vi "Execute_Circle_v1.vi"(0 "Resolution":i32=20, 1 "Speed":i32, 2 "x-disp":sgl[](array[numeric]), 3 "y-disp":sgl[](array[numeric]), 4 "GPIB Address":u8=6 max=100) -> (5 "x-position":i32, 6 "y-position":i32, 7 "Status":bool)   [LabVIEW 2010]
uses:
  <vilib>/express/express arith-compare/Formula/XNode/ExpressFormulaBlockNode.xnode
panel:
  out "XY Graph":T1(graph)
  in  "y-disp read":i32[](array[numeric])
  in  "x-disp read":i32[](array[numeric])
  # "Inputs"
  # "Outputs"
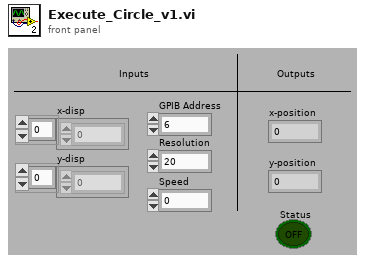
[diagram p1: front panel]
types:
  T1 = cluster{"x-disp read":i32[], "y-disp read":i32[]}
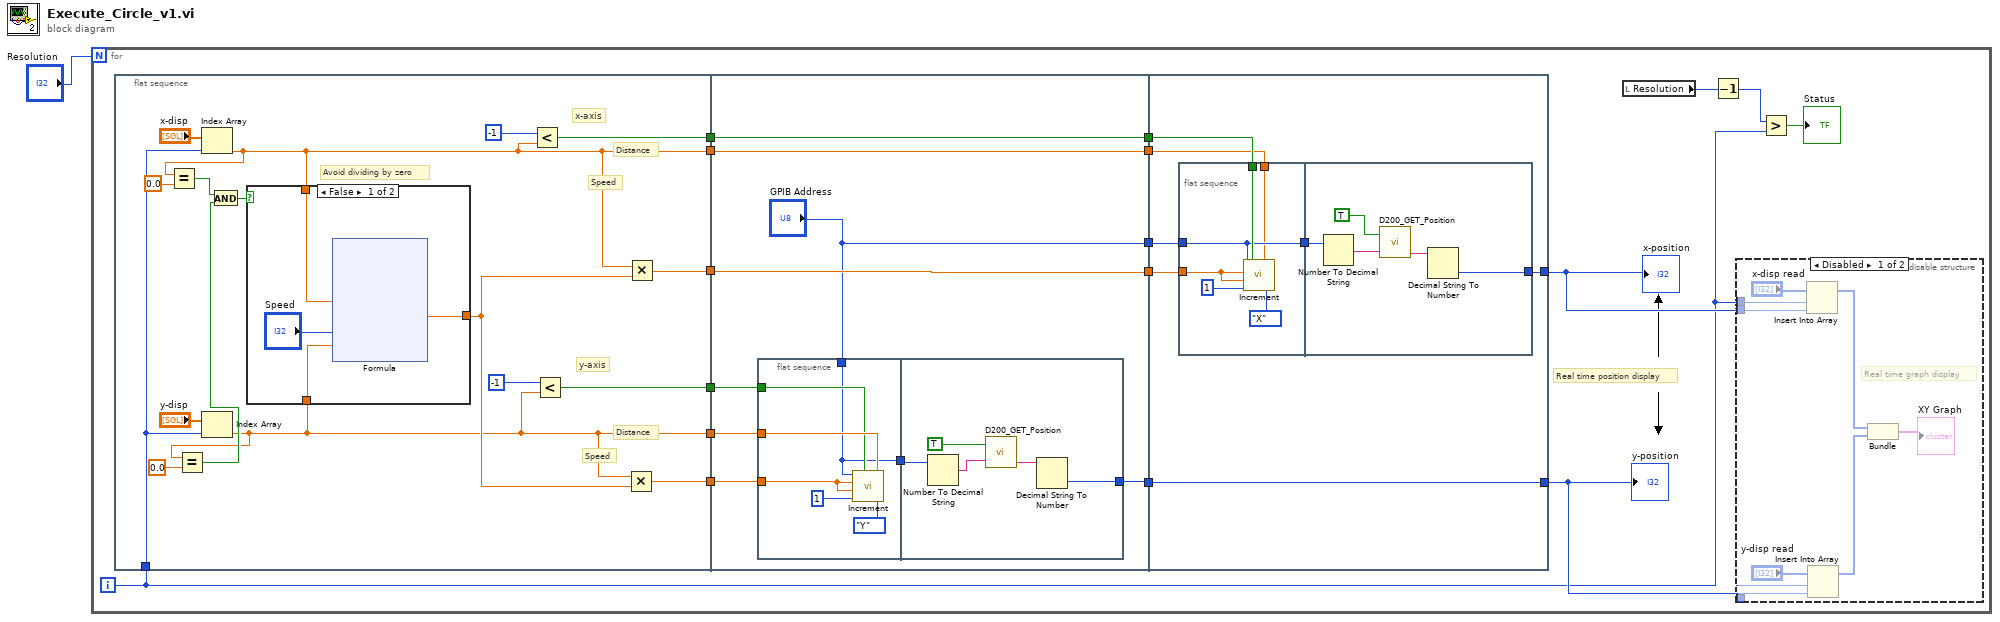
[diagram p0: block diagram]
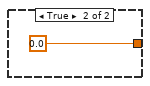
[diagram p3: hidden frame]
diagram:
  n1 = for {
    N: "Resolution" -> [_]
    i -> [w5]
    # "Real time position display"
    n2 = flat-sequence {
      tunnel: [w28] -> w18
      tunnel: [w41] -> w17
      tunnel: [w27] -> w16
      tunnel: [w40] -> w15
      tunnel: w5 -> [w35]
      tunnel: [w38] -> w14
      tunnel: [w39] -> w13
      tunnel: w18 -> [w61]
      tunnel: w17 -> [w64]
      tunnel: w16 -> [w68]
      tunnel: w15 -> [w67]
      tunnel: w14 -> [w69]
      tunnel: w13 -> [w63]
      tunnel: [w66] -> w12
      tunnel: [w63] -> w11
      tunnel: [w64] -> w10
      tunnel: ["GPIB Address"] -> w7
      tunnel: [w61] -> w6
      tunnel: [w87] -> w8
      tunnel: w12 -> [w87]
      tunnel: w11 -> [w84]
      tunnel: w10 -> [w83]
      tunnel: [w82] -> w9
      tunnel: w7 -> [w85]
      tunnel: w6 -> [w81]
      frame #0 {
        # "Avoid dividing by zero"
        # "y-axis"
        # "x-axis"
        # "Speed"
        # "Distance"
        # "Speed"
        # "Distance"
        n3 = Index Array(array="x-disp", index=w35) -> (element=w28:sgl)
        n4 = Equal?(x=w28, y=sgl 0.0) -> (x = y?=w32:bool)
        n5 = Index Array(array="y-disp", index=w35) -> (element=w27:sgl)
        n6 = Equal?(x=w27, y=sgl 0.0) -> (x = y?=w31:bool)
        n7 = And(x=w32, y=w31) -> (x .and. y?=w30:bool)
        n8 = case shown="False" w30 {
          tunnel: [w44 sgl 0.0] -> w29
          tunnel: w28 -> [w46 _]
          tunnel: w27 -> [w45 _]
          frame False {
            n9 = xnode "Formula"("X1"=w46, "X2"="Speed", "X3"=w45) -> ("Result"=w44:sgl)  [unwired: 1 in, 1 out]
          }
          frame True {
          }
        }
        n10 = Less?(x=-1, y=w28) -> (x < y?=w41:bool)
        n11 = Less?(x=-1, y=w27) -> (x < y?=w40:bool)
        n12 = Multiply(x=w27, y=w29) -> (x*y=w38:sgl)
        n13 = Multiply(x=w28, y=w29) -> (x*y=w39:sgl)
      }
      frame #1 {
        n14 = flat-sequence {
          tunnel: w69 -> [w75]
          tunnel: w68 -> [w74]
          tunnel: w67 -> [w73]
          tunnel: [w70] -> w65
          tunnel: "GPIB Address" -> [w70]
          tunnel: [w77] -> w66
          tunnel: w65 -> [w76]
          frame #0 {
            n15 = call "Increment.vi"("GPIB_Addr"=w70, "F Speed"=w75, "L Speed"=w75, "Rate"=u16 1, "CCW 3"=w73, "Distance"=w74, "Axis"=enum16{"X", "Y", "Z", "U", "V", "W"}."Y") -> ()
          }
          frame #1 {
            n16 = Number To Decimal String(number=w76) -> (decimal integer string=w79:string)  [unwired: 1 in]
            n17 = call "D200_GET_Position.vi"("Permission"=TRUE, "GPIB Addr"=w79) -> ("Current position"=w78:string)  [unwired: 2 out]
            n18 = Decimal String To Number(string=w78) -> (number=w77:i32)  [unwired: 2 in, 1 out]
          }
        }
      }
      frame #2 {
        n19 = flat-sequence {
          tunnel: w83 -> [w93]
          tunnel: w84 -> [w92]
          tunnel: w85 -> [w90]
          tunnel: [w90] -> w86
          tunnel: w81 -> [w88]
          tunnel: [w95] -> w82
          tunnel: w86 -> [w94]
          frame #0 {
            n20 = call "Increment.vi"("GPIB_Addr"=w90, "F Speed"=w92, "L Speed"=w92, "Rate"=u16 1, "CCW 3"=w93, "Distance"=w88, "Axis"=enum16{"X", "Y", "Z", "U", "V", "W"}."X") -> ()
          }
          frame #1 {
            n21 = Number To Decimal String(number=w94) -> (decimal integer string=w97:string)  [unwired: 1 in]
            n22 = call "D200_GET_Position.vi"("Permission"=TRUE, "GPIB Addr"=w97) -> ("Current position"=w96:string)  [unwired: 2 out]
            n23 = Decimal String To Number(string=w96) -> (number=w95:i32)  [unwired: 2 in, 1 out]
          }
        }
      }
    }
    n24 = local read "Resolution"() -> (w3:i32)
    n25 = Decrement(x=w3) -> (x-1=w2:i32)
    n26 = disable-structure shown="Disabled" {
      disable-tunnel: w5 -> [w26 _]
      disable-tunnel: w9 -> [w25 _]
      disable-tunnel: w8 -> [w24 _]
      frame Disabled {
        # "Real time graph display"
        n27 = Insert Into Array(array="x-disp read", index=w26, new element=w25) -> (w21:i32[])
        n28 = Insert Into Array(array="y-disp read", index=w26, new element=w24) -> (w20:i32[])
        n29 = Bundle("x-disp read"=w21, "y-disp read"=w20) -> (→"XY Graph":T1)  [unwired: 1 in]
      }
      frame Enabled {
      }
    }
    n30 = Greater?(x=w2, y=w5) -> (0:→"Status":bool)
    "x-position" <- w9
    "y-position" <- w8
  }
